vi "myRIO_BRig_RT_arrTrig_Select_laserOn_l2.vi"() -> (2 "output_arrTrig_Select_laserOn_l2":i32)   [LabVIEW 2014]
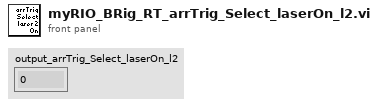
[diagram p1: front panel]
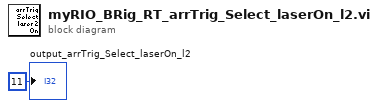
[diagram p0: block diagram]
diagram:
  "output_arrTrig_Select_laserOn_l2" <- 11
